vi "Is Actuator Stopped.vi"(1 "Actuator Stopped Threshold":dbl(slide)=0.014715719063545152 scale=0.0..0.2, 2 "Voltage Delta":dbl=0.005140088999999737) -> (0 "Stopped?":bool=TRUE)   [LabVIEW 2012]
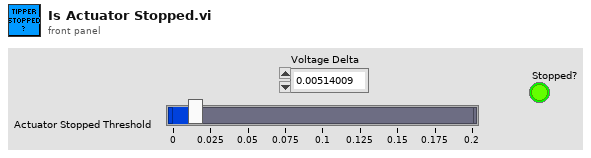
[diagram p1: front panel]
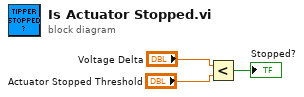
[diagram p0: block diagram]
diagram:
  n1 = Less?(x="Voltage Delta", y="Actuator Stopped Threshold") -> (x < y?=→"Stopped?":bool)
